vi "数值条件结构.vi"() -> ()   [LabVIEW 2022 SP3]
doc: "本VI是为《我和LabVIEW》一书编写的示例。\n关于本书的介绍请参考网页：\nhttp://ruanqizhen.spaces.live.com/blog/cns!5852D4F797C53FB6!4310.entry"
panel:
  in  "数值":i32
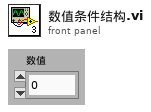
[diagram p1: front panel]
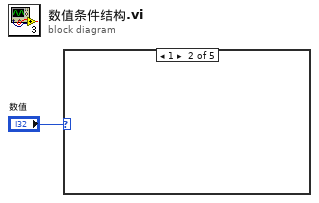
[diagram p0: block diagram]
diagram:
  n1 = case shown="1" "数值" {
    frame 0, Default {
    }
    frame 1 {
    }
    frame 2, 4, 6 {
    }
    frame 7..11 {
    }
    frame 12.. {
      # "所有大于等于12的整数"
    }
  }
